vi "Read PowerSV refnum.vi"(8 "error in (no error)":errorcluster, 11 "UniStableShutter in":refnum<class "UniStableShutter.lvclass">) -> (0 "error out":errorcluster, 2 "PowerSV refnum":refnum<k21>, 3 "UniStableShutter out":refnum<class "UniStableShutter.lvclass">)   [LabVIEW 2016, in "UniStableShutter.lvclass"]
uses:
  UniStableShutter.lvclass
  UniStableShutter.lvclass/UniStableShutter.ctl
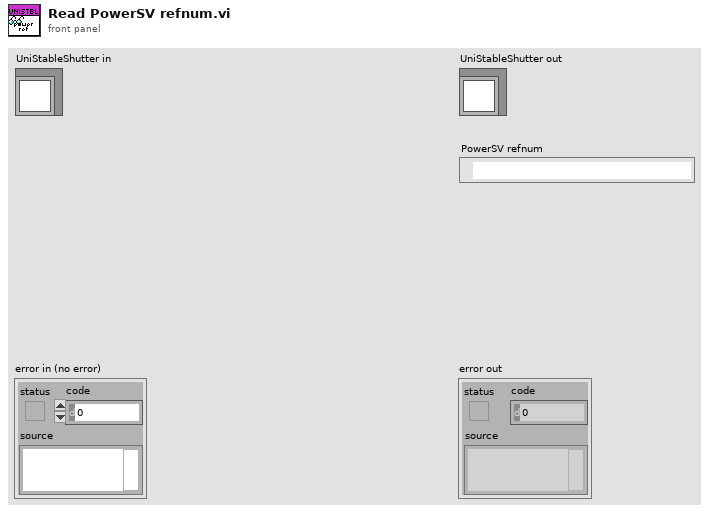
[diagram p1: front panel]
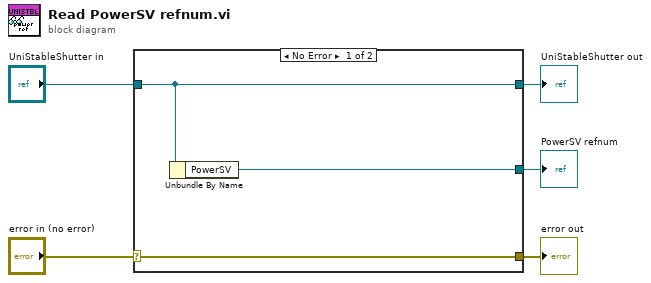
[diagram p0: block diagram]
diagram:
  n1 = case shown="No Error" "error in (no error)" {
    selector: "error in (no error)" -> [w8 w9]
    tunnel: [w8 w9] -> w4
    tunnel: [w7 w10] -> w2
    tunnel: "UniStableShutter in" -> [w7 w10]
    tunnel: [w6 _] -> w1
    frame No Error {
      n2 = Unbundle By Name(w7) -> ("PowerSV"=w6:refnum<k21>)
    }
    frame Error {
    }
  }
  "error out" <- w4
  "UniStableShutter out" <- w2
  "PowerSV refnum" <- w1
